vi "Write Config File Handle.vi"(10 "Session Handle":T1, 11 "Abstract Controller in":refnum<class "Abstract Controller.lvclass">) -> (3 "Abstract Controller out":refnum<class "Abstract Controller.lvclass">)   [LabVIEW 2016, in "_Controllers.lvlib" / "Abstract Controller.lvclass"]
uses:
  Abstract Controller.lvclass
  Configurations/Configurations.lvclass
  Configurations/Typedefs/Session Handle.ctl
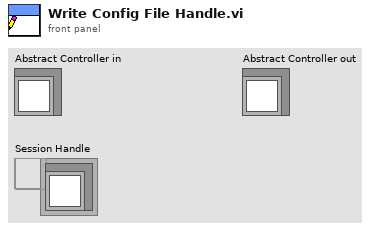
[diagram p1: front panel]
types:
  T1 = typedef "Configurations.lvlib/Configurations.lvclass/Session Handle.ctl" = refnum<data-value>
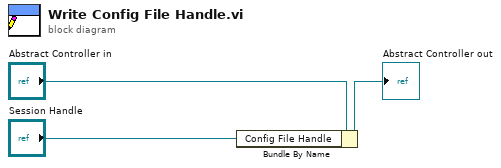
[diagram p0: block diagram]
diagram:
  n1 = Bundle By Name(cluster="Abstract Controller in", "Config File Handle"="Session Handle") -> (→"Abstract Controller out":refnum<class "Abstract Controller.lvclass">)
